vi "getAllProperties.vi"(8 "error in (no error)":errorcluster, 11 "IPropertyObject in":refnum<class "IPropertyObject.lvclass">) -> (0 "error out":errorcluster, 2 "All Properties out":refnum<class "IProperty.lvclass">[](array[class]), 3 "IPropertyObject out":refnum<class "IPropertyObject.lvclass">)   [LabVIEW 2022 SP3, in "openDAQ.lvlib" / "IBaseObject.lvlib" / "IPropertyObject.lvlib" / "IPropertyObject.lvclass"]
uses:
  <instrlib>/openDAQ/Public/Classes/IPropertyObject/IPropertyObject.lvclass
  <instrlib>/openDAQ/Public/Classes/IPropertyObject/IPropertyObject.lvclass/IPropertyObject.ctl
  <instrlib>/openDAQ/Public/Classes/daqCoreTypes/IList/IList.lvclass
  <instrlib>/openDAQ/Binaries/Windows/x86/copendaq32.dll
  <instrlib>/openDAQ/Public/Classes/daqCoreTypes/IList/Polymorphic/getList/getPropertyList.vi
  <instrlib>/openDAQ/Public/Classes/IProperty/IProperty.lvclass
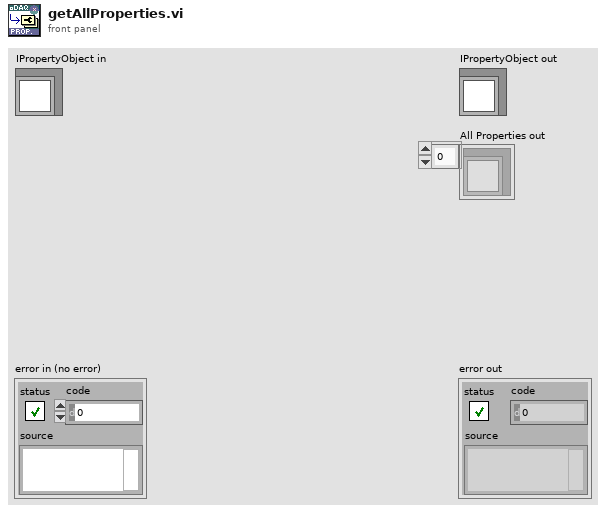
[diagram p1: front panel]
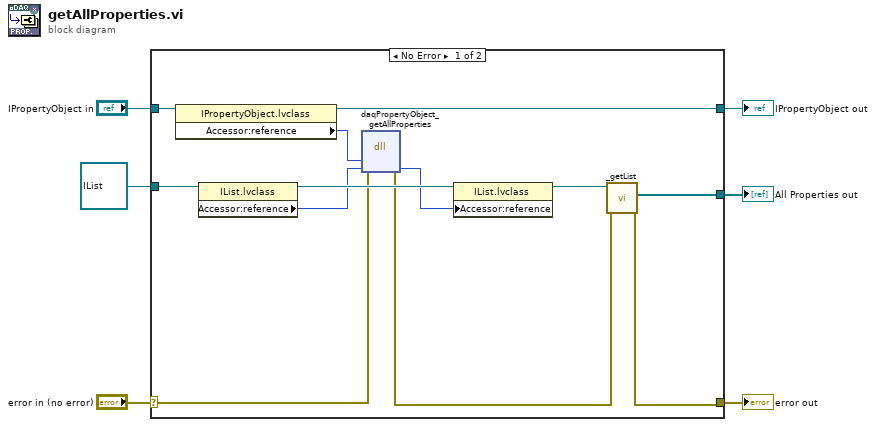
[diagram p0: block diagram]
diagram:
  n1 = case shown="No Error" "error in (no error)" {
    selector: "error in (no error)" -> [w11 w20]
    tunnel: [w7 w20] -> w5
    tunnel: [w16 w19] -> w3
    tunnel: "IPropertyObject in" -> [w17 w19]
    tunnel: refnum<class "IList.lvclass"> refnum ("openDAQ.lvlib:daqCoreTypes.lvlib:IList.lvclass") -> [w14 _]
    tunnel: [w9 _] -> w1
    frame No Error {
      n2 = property class="IPropertyObject.lvclass"(reference=w17) -> (reference out=w16:refnum<class "IPropertyObject.lvclass">, "Accessor:reference"=w15:i64)  [unwired: 1 in, 1 out]
      n3 = property class="IList.lvclass"(reference=w14) -> (reference out=w18:refnum<class "IList.lvclass">, "Accessor:reference"=w13:i64)  [unwired: 1 in, 1 out]
      n4 = dll-call lib="C:/Program Files (x86)/National Instruments/LabVIEW 2022/instr.lib/openDAQ/Binaries/Windows/x86/copendaq*.*" fn="daqPropertyObject_getAllProperties"(error in=w11, "propertyObject"=w15, "allProperties"=w13) -> (error out=w8:errorcluster, "allProperties"=w12:i64)  [unwired: 4 in, 1 out]
      n5 = property class="IList.lvclass"(reference=w18, "Accessor:reference"=w12) -> (reference out=w10:refnum<class "IList.lvclass">)  [unwired: 1 in, 1 out]
      n6 = call-poly <instrlib>:"_getList.vi"("error in (no error)"=w8, "IList in"=w10) -> ("error out"=w7:errorcluster, "Properties out"=w9:refnum<class "IProperty.lvclass">[])  [unwired: 8 in]
    }
    frame Error {
    }
  }
  "error out" <- w5
  "IPropertyObject out" <- w3
  "All Properties out" <- w1
